vi "Build G Object From Btye Stream.vi"(8 "error in (no error)":errorcluster, 9 "Byte Stream in":u8[](array[numeric]), 10 "Type Name":string, 11 "TwinCAT ADS in":refnum<class "TwinCAT ADS.lvclass">) -> (0 "error out":errorcluster, 1 "Byte Stream out":u8[](array[numeric]), 2 "Value":variant, 3 "TwinCAT ADS out":refnum<class "TwinCAT ADS.lvclass">)   [LabVIEW 2018, in "TwinCAT ADS.lvclass"]
uses:
  TwinCAT ADS.lvclass
  TwinCAT.Ads
  PLC Primitive Byte Stream to G Object.vi/dd5e40b3-f89d-44d0-b911-1f2dc1f1e391.vi
  PLC Primitive Byte Stream to G Object.vi/9a8c356b-cf55-4838-9201-0532b80217b2.vi
  PLC Primitive Byte Stream to G Object.vi/06482052-d1f9-4f29-aca9-908031c6a69f.vi
  PLC Primitive Byte Stream to G Object.vi/b9242781-96b0-446e-9150-452b1084ed54.vi
  PLC Primitive Byte Stream to G Object.vi/5fbe6976-0b86-40a2-b7b6-3748894f0071.vi
  PLC Primitive Byte Stream to G Object.vi/c4de1741-fffd-4fed-ba25-d7b4acbf0555.vi
  PLC Primitive Byte Stream to G Object.vi/20356124-05d2-4a04-a5d1-e69adc4c58c2.vi
  PLC Primitive Byte Stream to G Object.vi/67ddb754-0fbe-43d9-9e61-34d6659124ef.vi
  PLC Primitive Byte Stream to G Object.vi/e3d41cb3-d20e-45e9-8252-e41884a8f4d0.vi
  PLC Primitive Byte Stream to G Object.vi/46ba2a54-cc07-4222-9a0e-bd972edfcef0.vi
  PLC Primitive Byte Stream to G Object.vi/6b416cf7-30dc-48a3-9278-9d800f443678.vi
  PLC Primitive Byte Stream to G Object.vi/5857d013-9824-4299-a2d7-53efdc0d26c5.vi
  PLC Primitive Byte Stream to G Object.vi/006b0e7e-7e80-41f3-be4e-1f3da8479fae.vi
  PLC Primitive Byte Stream to G Object.vi/28d9c90b-5f2a-4c58-95e2-5fc46303b0fd.vi
  PLC Primitive Byte Stream to G Object.vi/99b7bc4a-962e-4818-aa5d-444f23f83b11.vi
  PLC Primitive Byte Stream to G Object.vi/8b7c42c8-9170-4542-8f35-15cbeddc22cb.vi
  PLC Primitive Byte Stream to G Object.vi/65a091fa-0bd2-4a35-ae2b-3fa5e90d1994.vi
  PLC Primitive Byte Stream to G Object.vi/4b7d3a7d-7f1b-46f0-9357-48cb72148c56.vi
  PLC Primitive Byte Stream to G Object.vi/b431183c-2ad5-4c6d-9bfa-a53b18913682.vi
  PLC Primitive Byte Stream to G Object.vi/30c6c28a-53c3-4e33-80b1-b22f521e1f67.vi
  PLC Struct Byte Stream to Data String.vi
  PLC Array Byte Stream to Data String.vi
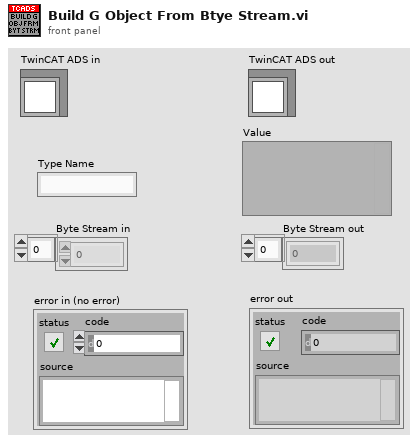
[diagram p1: front panel]
types:
  T1 = typedef "TwinCAT ADS.lvclass/PLC Type.ctl" = enum16{"UNDEFINED", "INT", "DINT", "REAL", "LREAL", "SINT", "BYTE", "UINT", "UDINT", "LINT", "ULINT", "STRING", "WSTRING", "BOOL", "TIME", "LTIME", "DATE", "DT", "TOD", "ARRAY", "JAGGED ARRAY", "STRUCT", "FUNCTION BLOCK", "POINTER", "USER DEFINED"}
  T2 = typedef "TwinCAT ADS.lvclass/PLC Sub-Item Type Descriptor.ctl" = cluster{"PLC Type":T1, "Offset":i32, "Byte Size":i32, "[Sub-Item/Array Type Descriptor]":variant[]}
  T3 = typedef "TwinCAT ADS.lvclass/PLC Array Type Descriptor.ctl" = cluster{"Fundamental PLC Type":T1, "Fundamental Type Byte Size":i32, "Item Count":i32, "Dimension Lengths":i32[], "Sub-Item Type Descriptor":variant}
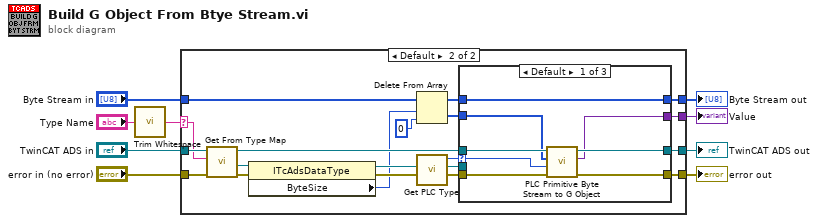
[diagram p0: block diagram]
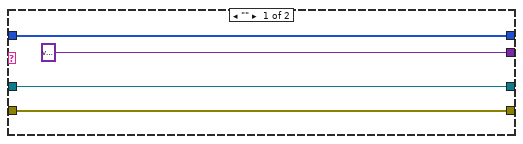
[diagram p2: hidden frame]
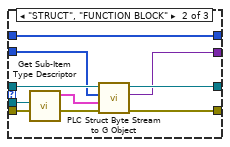
[diagram p3: hidden frame]
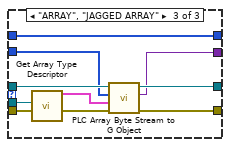
[diagram p4: hidden frame]
diagram:
  n1 = call <vilib>:"Trim Whitespace.vi"("string"="Type Name") -> ("trimmed string"=w1:string)  [unwired: 1 in]
  n2 = case shown="Default" w1 {
    selector: w1 -> [_ w26]
    tunnel: [variant ("Value") w33] -> w9
    tunnel: [w11 w32] -> w8
    tunnel: [w10 w31] -> w7
    tunnel: [w13 w30] -> w6
    tunnel: "error in (no error)" -> [w10 w29]
    tunnel: "TwinCAT ADS in" -> [w11 w28]
    tunnel: "Byte Stream in" -> [w13 w27]
    frame "" {
    }
    frame Default {
      n3 = call "Get From Type Map.vi"("error in (no error)"=w29, "Type Name"=w26, "TwinCAT ADS in"=w28) -> ("error out"=w17:errorcluster, ".NET AdsDataType"=w15:refnum<k24>, "TwinCAT ADS out"=w16:refnum<class "TwinCAT ADS.lvclass">)  [unwired: 6 in]
      n4 = property class="ITcAdsDataType"(reference=w15, error in=w17) -> (reference out=w21:refnum<k24>, error out=w22:errorcluster, "ByteSize"=w14:i32)
      n5 = Delete From Array(array=w27, length=w14, index=0) -> (deleted portion=w23:u8[], array with subset deleted=w24:u8[])
      n6 = call "Get PLC Type.vi"("error in (no error)"=w22, ".NET AdsDataType in"=w21) -> ("error out"=w20:errorcluster, ".NET AdsDataType"=w19:refnum<k24>, "PLC Type"=w18:T1)  [unwired: 7 in]
      n7 = case shown="Default" w18 {
        selector: w18 -> [w34 _ _]
        tunnel: w20 -> [w35 w50 w55]
        tunnel: w19 -> [_ w49 w54]
        tunnel: w24 -> [w37 w51 w61]
        tunnel: [w40 w44 w58] -> w31
        tunnel: [w39 w42 w56] -> w33
        tunnel: w16 -> [w38 w48 w60]
        tunnel: [w41 w43 w57] -> w32
        tunnel: [w37 w51 w61] -> w30
        tunnel: w23 -> [w36 w47 w59]
        frame Default {
          n8 = call "PLC Primitive Byte Stream to G Object.vi"("error in (no error)"=w35, "PLC Type"=w34, "Byte Stream"=w36, "TwinCAT ADS in"=w38) -> ("error out"=w40:errorcluster, "Value"=w39:variant, "TwinCAT ADS out"=w41:refnum<class "TwinCAT ADS.lvclass">)  [unwired: 5 in]
        }
        frame "STRUCT", "FUNCTION BLOCK" {
          n9 = call "Get Sub-Item Type Descriptor.vi"("error in (no error)"=w50, ".NET AdsDataType"=w49) -> ("error out"=w45:errorcluster, "[Sub-Item Type Descriptor]"=w46:T2[])  [unwired: 7 in, 1 out]
          n10 = call "PLC Struct Byte Stream to G Object.vi"("error in (no error)"=w45, "[Sub-Item Type Information]"=w46, "Byte Stream"=w47, "TwinCAT ADS in"=w48) -> ("error out"=w44:errorcluster, "Value"=w42:variant, "TwinCAT ADS out"=w43:refnum<class "TwinCAT ADS.lvclass">)  [unwired: 5 in]
        }
        frame "ARRAY", "JAGGED ARRAY" {
          n11 = call "Get Array Type Descriptor.vi"("error in (no error)"=w55, ".NET AdsDataType"=w54) -> ("error out"=w53:errorcluster, "Array Type Descriptor"=w52:T3)  [unwired: 7 in, 1 out]
          n12 = call "PLC Array Byte Stream to G Object.vi"("error in (no error)"=w53, "Array Type Descriptor"=w52, "Byte Stream"=w59, "TwinCAT ADS in"=w60) -> ("error out"=w58:errorcluster, "Value"=w56:variant, "TwinCAT ADS out"=w57:refnum<class "TwinCAT ADS.lvclass">)  [unwired: 5 in]
        }
      }
    }
  }
  "Value" <- w9
  "error out" <- w7
  "TwinCAT ADS out" <- w8
  "Byte Stream out" <- w6
